vi "Unbenannt 1.vi"() -> ()   [LabVIEW 2020, in "EPA 1065.lvlib" / "Chiller NO2 1065-376.lvlib"]
uses:
  Chiller NO2 1065-376.lvlib
panel:
  out "Array":bool[](array[boolean])
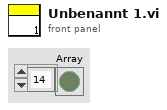
[diagram p1: front panel]
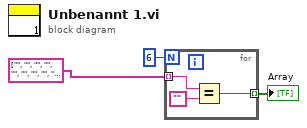
[diagram p0: block diagram]
diagram:
  n1 = for {
    N: 6 -> [_]
    tunnel: string[] ["", "", "", "", "", "", "", "", "", "", "0"] -> [w6] mode=indexing
    tunnel: [w4] -> w1 mode=indexing
    n2 = Equal?(x=w6, y="") -> (x = y?=w4:bool)
  }
  "Array" <- w1
